vi "Get Many Attributes Priv.vi"(0 "Tree Dictionary In":variant, 5 "Unique ID":string, 7 "Attribute Names":string[](array[string]), 11 "error in":errorcluster) -> (4 "Tree Dictionary Out":variant, 6 "Attribute Names":string[](array[string]), 8 "Found?":bool[](array[boolean]), 10 "Attribute Values":variant[](array[variant]), 13 "Data IDs":string[](array[string]), 15 "error out":errorcluster)   [LabVIEW 2017, in "Tree API.lvlib" / "Tree.lvclass"]
uses:
  Tree.lvclass
  <vilib>/ErrorRing/Error Ring.xnode
  Typedefs/Tree Cluster.ctl
  <vilib>/Utility/error.llb/Error Cluster From Error Code.vi
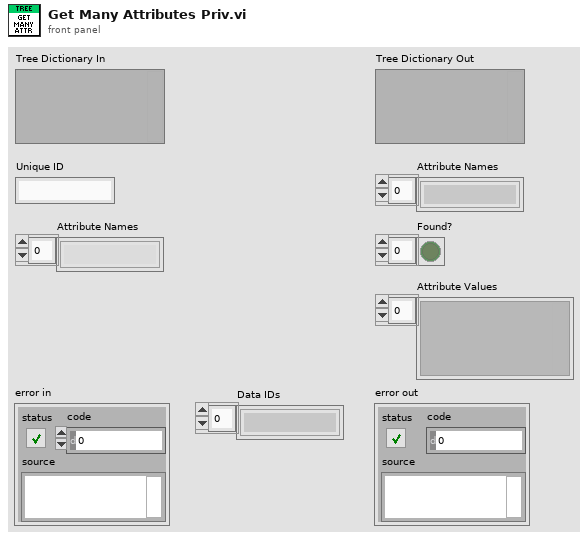
[diagram p1: front panel]
types:
  T1 = typedef "Tree API.lvlib/Tree.lvclass/Tree Cluster.ctl" = cluster{"Unique ID":string, "Parent ID":string, "Child IDs":string[], "Name":string, "MetaData":string, "Data IDs":string[]}
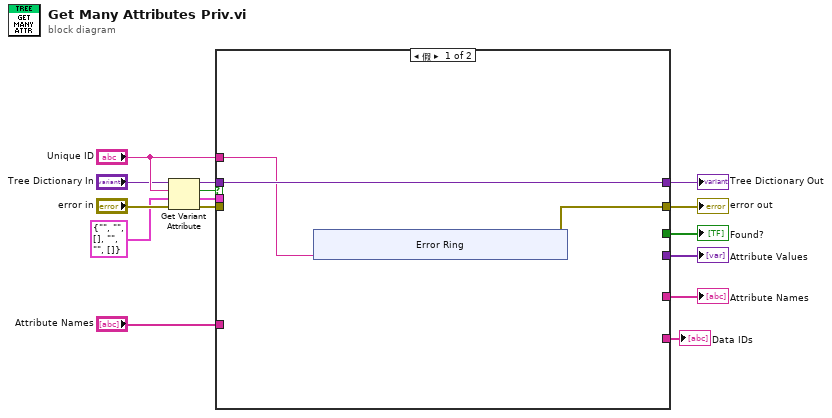
[diagram p0: block diagram]
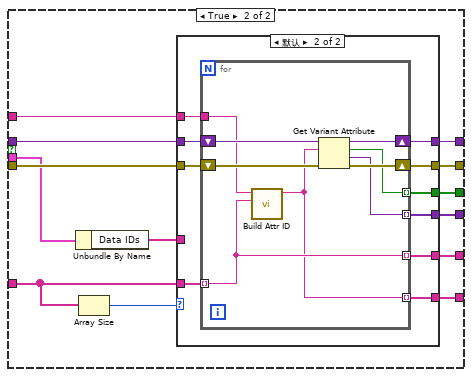
[diagram p2: hidden frame]
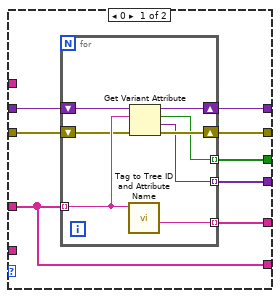
[diagram p3: hidden frame]
diagram:
  n1 = Get Variant Attribute(Variant="Tree Dictionary In", name="Unique ID", default value (empty Variant)=T1 {"Unique ID"="", "Parent ID"="", "Child IDs"=[], "Name"="", "MetaData"="", "Data IDs"=[]} ("Cluster of class private data"), error in="error in") -> (duplicate Variant=w12:variant, found=w13:bool, value=w14:T1, error out=w10:errorcluster)
  n2 = case shown="假" w13 {
    tunnel: [w17 w37] -> w8
    tunnel: [w18 w28] -> w9
    tunnel: w10 -> [_ w38]
    tunnel: w12 -> [w18 w29]
    tunnel: w14 -> [_ w34]
    tunnel: "Unique ID" -> [w16 w27]
    tunnel: [_ w36] -> w3
    tunnel: [_ w35] -> w5
    tunnel: "Attribute Names" -> [_ w32]
    tunnel: [_ w30] -> w2
    tunnel: [_ w26] -> w1
    frame False {
      n3 = xnode "Error Ring"("参数 0"=w16) -> ("错误输出"=w17:errorcluster)
    }
    frame True {
      n4 = Unbundle By Name(w34) -> ("Data IDs"=w33:string[])
      n5 = Array Size(array=w32) -> (size(s)=w31:i32)
      n6 = case shown="默认" w31 {
        tunnel: w38 -> [w44 w64]
        tunnel: [w43 w63] -> w37
        tunnel: [w40 w62] -> w36
        tunnel: [w41 w61] -> w35
        tunnel: w33 -> [w39 _]
        tunnel: w32 -> [_ w60]
        tunnel: [w45 w59] -> w30
        tunnel: w29 -> [w46 w58]
        tunnel: [w42 w56] -> w28
        tunnel: w27 -> [_ w57]
        tunnel: [w39 w55] -> w26
        frame 0 {
          n7 = for {
            shift-right: [w53] -> w42
            shift-left: w46 -> [w54]
            tunnel: w39 -> [w52] mode=indexing
            tunnel: [w51] -> w45 mode=indexing
            shift-right: [w49] -> w43
            shift-left: w44 -> [w50]
            tunnel: [w48] -> w41 mode=indexing
            tunnel: [w47] -> w40 mode=indexing
            n8 = call "Tag to Tree ID and Attribute Name.vi"("Tag"=w52) -> ("Attribute Name"=w51:string)  [unwired: 8 in, 2 out]
            n9 = Get Variant Attribute(Variant=w54, name=w52, error in=w50) -> (duplicate Variant=w53:variant, found=w47:bool, value=w48:variant, error out=w49:errorcluster)  [unwired: 1 in]
          }
        }
        frame Default {
          n10 = for {
            tunnel: [w71] -> w62 mode=indexing
            tunnel: [w70] -> w61 mode=indexing
            shift-right: [w72] -> w63
            shift-left: w64 -> [w73]
            shift-right: [w69] -> w56
            shift-left: w58 -> [w68]
            tunnel: w60 -> [w66] mode=indexing
            tunnel: [w66] -> w59 mode=indexing
            tunnel: w57 -> [w67]
            tunnel: [w65] -> w55 mode=indexing
            n11 = call "Build Attr ID.vi"("Attr Name"=w66, "Unique ID"=w67) -> ("Attr ID Out"=w65:string)  [unwired: 9 in]
            n12 = Get Variant Attribute(Variant=w68, name=w65, error in=w73) -> (duplicate Variant=w69:variant, found=w71:bool, value=w70:variant, error out=w72:errorcluster)  [unwired: 1 in]
          }
        }
      }
    }
  }
  "Tree Dictionary Out" <- w9
  "error out" <- w8
  "Attribute Values" <- w5
  "Found?" <- w3
  "Attribute Names" <- w2
  "Data IDs" <- w1
